vi "Mod3 9205 Read.vi"(10 "error in":errorcluster) -> (2 "error out":errorcluster, 3 "data out":fxp<+/-,26,5>[](array[numeric]))   [LabVIEW 2015]
uses:
  <vilib>/rvi/eio/common/nirviEmuTemplateMethod_errors.vi
  <vilib>/eio/EIONode/EIONode.xnode
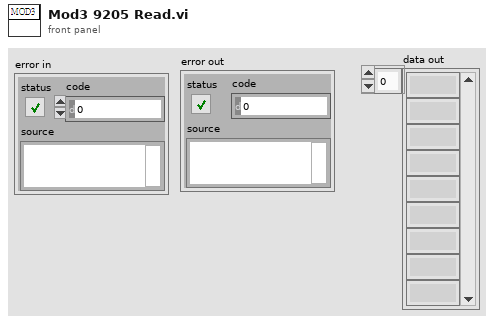
[diagram p1: front panel]
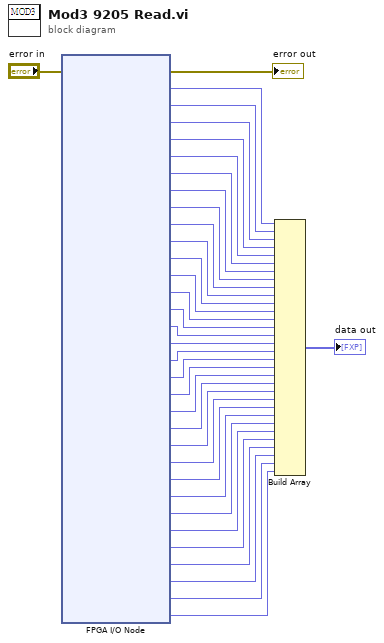
[diagram p0: block diagram]
diagram:
  n1 = xnode "FPGA I/O Node"("error in"="error in") -> ("error out"=→"error out":errorcluster, "Mod3/AI0"=w35:fxp<+/-,26,5>, "Mod3/AI1"=w34:fxp<+/-,26,5>, "Mod3/AI2"=w33:fxp<+/-,26,5>, "Mod3/AI3"=w32:fxp<+/-,26,5>, "Mod3/AI4"=w31:fxp<+/-,26,5>, "Mod3/AI5"=w30:fxp<+/-,26,5>, "Mod3/AI6"=w29:fxp<+/-,26,5>, "Mod3/AI7"=w28:fxp<+/-,26,5>, "Mod3/AI8"=w27:fxp<+/-,26,5>, "Mod3/AI9"=w26:fxp<+/-,26,5>, "Mod3/AI10"=w25:fxp<+/-,26,5>, "Mod3/AI11"=w24:fxp<+/-,26,5>, "Mod3/AI12"=w23:fxp<+/-,26,5>, "Mod3/AI13"=w22:fxp<+/-,26,5>, "Mod3/AI14"=w21:fxp<+/-,26,5>, "Mod3/AI15"=w20:fxp<+/-,26,5>, "Mod3/AI16"=w19:fxp<+/-,26,5>, "Mod3/AI17"=w18:fxp<+/-,26,5>, "Mod3/AI18"=w17:fxp<+/-,26,5>, "Mod3/AI19"=w16:fxp<+/-,26,5>, "Mod3/AI20"=w15:fxp<+/-,26,5>, "Mod3/AI21"=w14:fxp<+/-,26,5>, "Mod3/AI22"=w13:fxp<+/-,26,5>, "Mod3/AI23"=w12:fxp<+/-,26,5>, "Mod3/AI24"=w11:fxp<+/-,26,5>, "Mod3/AI25"=w10:fxp<+/-,26,5>, "Mod3/AI26"=w9:fxp<+/-,26,5>, "Mod3/AI27"=w8:fxp<+/-,26,5>, "Mod3/AI28"=w7:fxp<+/-,26,5>, "Mod3/AI29"=w6:fxp<+/-,26,5>, "Mod3/AI30"=w5:fxp<+/-,26,5>, "Mod3/AI31"=w4:fxp<+/-,26,5>)  [unwired: 32 in, 32 out]
  n2 = Build Array(w35, w34, w33, w32, w31, w30, w29, w28, w27, w26, w25, w24, w23, w22, w21, w20, w19, w18, w17, w16, w15, w14, w13, w12, w11, w10, w9, w8, w7, w6, w5, w4) -> (→"data out":fxp<+/-,26,5>[])
